vi "StopAcquisitionResponseMessage_Parse.vi"(8 "error in (no error)":errorcluster, 11 "message":variant) -> (0 "error out":errorcluster, 2 "Stop Acquisition Response":T1)   [LabVIEW 2017, in "CmsAcquisition.lvlib"]
uses:
  <vilib>/addons/InsightCM/Devices/Shared/Cms/CmsAcquisition/CmsAcquisition.lvlib
  <vilib>/addons/InsightCM/Devices/Shared/Cms/CmsAcquisition/controls/StopAcquisitionResponse.ctl
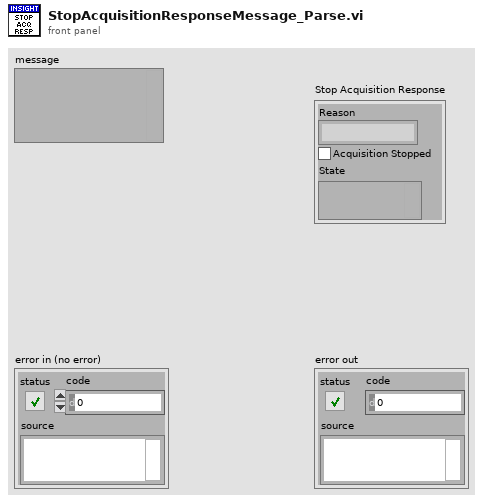
[diagram p1: front panel]
types:
  T1 = typedef "CmsAcquisition.lvlib/StopAcquisitionResponse.ctl" = cluster{"Reason":string, "Acquisition Stopped":bool, "State":variant}
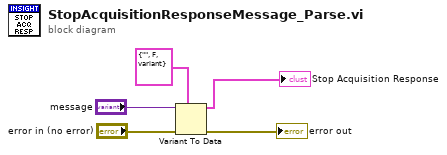
[diagram p0: block diagram]
diagram:
  n1 = Variant To Data(error in="error in (no error)", type=T1 {"Reason"="", "Acquisition Stopped"=FALSE, "State"=variant} ("Stop Acquisition Response"), Variant="message") -> (data=→"Stop Acquisition Response":T1, error out=→"error out":errorcluster)
